vi "ChooseManualPressuresChan3_4.vi"(7 "Manual Pressure In":dbl[](array[numeric]), 10 "Calibration Refs":T1, 11 "Set Pressures":dbl[][](array[numeric])=[[665.1538332158755, 622.4106177021335]]) -> (3 "Manual Pressure":dbl[](array[numeric]))   [LabVIEW 2016]
panel:
  # "supposed to find reasonable pressures to apply by default"
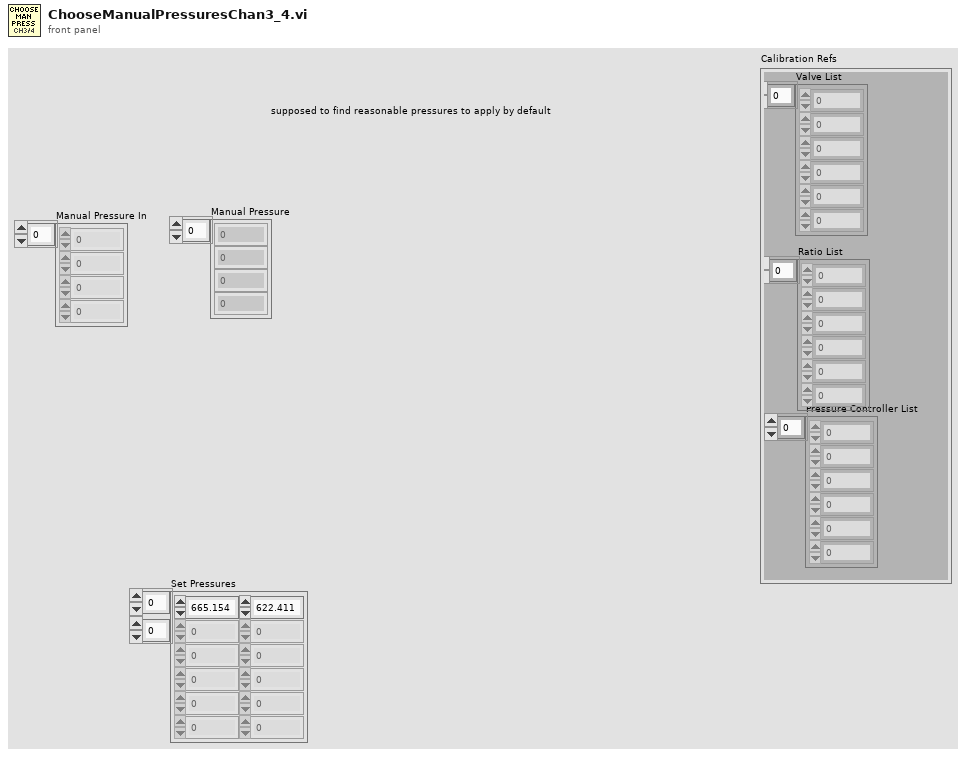
[diagram p1: front panel]
types:
  T1 = cluster{"Pressure Controller List":u8[], "Ratio List":dbl[], "Valve List":u16[]}
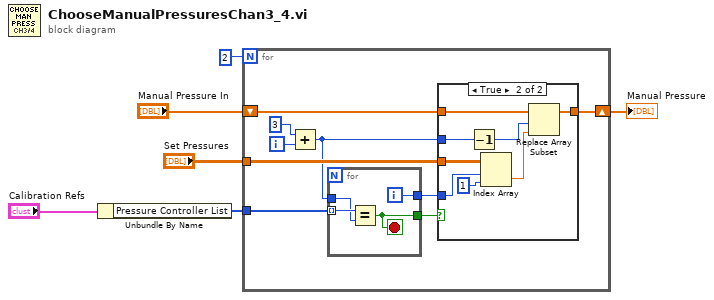
[diagram p0: block diagram]
diagram:
  n1 = Unbundle By Name("Calibration Refs") -> ("Pressure Controller List"=w1:u8[])
  n2 = for {
    N: 2 -> [_]
    tunnel: w1 -> [w15]
    tunnel: "Set Pressures" -> [w12]
    shift-right: [w9] -> w4
    shift-left: "Manual Pressure In" -> [w8]
    i -> [w14]
    n3 = Add(x=3, y=w14) -> (x+y=w10:i32)
    n4 = for {
      tunnel: w15 -> [w19] mode=indexing
      tunnel: w10 -> [w18]
      tunnel: [w17] -> w11
      tunnel: [w16] -> w7
      i -> [w17]
      stop <- w16 stop-if-true
      n5 = Equal?(x=w19, y=w18) -> (x = y?=w16:bool)
    }
    n6 = case shown="True" w7 {
      tunnel: w12 -> [_ w28]
      tunnel: w11 -> [_ w27]
      tunnel: w10 -> [_ w25]
      tunnel: [w20 w23] -> w9
      tunnel: w8 -> [w20 w22]
      frame False {
      }
      frame True {
        n7 = Decrement(x=w25) -> (x-1=w24:i32)
        n8 = Index Array(array=w28, index (row)=w27, index (col)=1 ("disabled index (col)")) -> (element=w26:dbl)
        n9 = Replace Array Subset(array=w22, new element=w26, index=w24) -> (w23:dbl[])
      }
    }
  }
  "Manual Pressure" <- w4
